vi "TRUE_Serial_GET.vi"() -> ()   [LabVIEW 2016]
uses:
  <vilib>/Instr/_visa.llb/VISA Configure Serial Port (Instr).vi
panel:
  out "Array":dbl[][](array[numeric])
  out "read buffer":string
  out "Cluster":T1
  in  "VISA resource name":refnum<visa-resource-name>
  in  "stop":bool
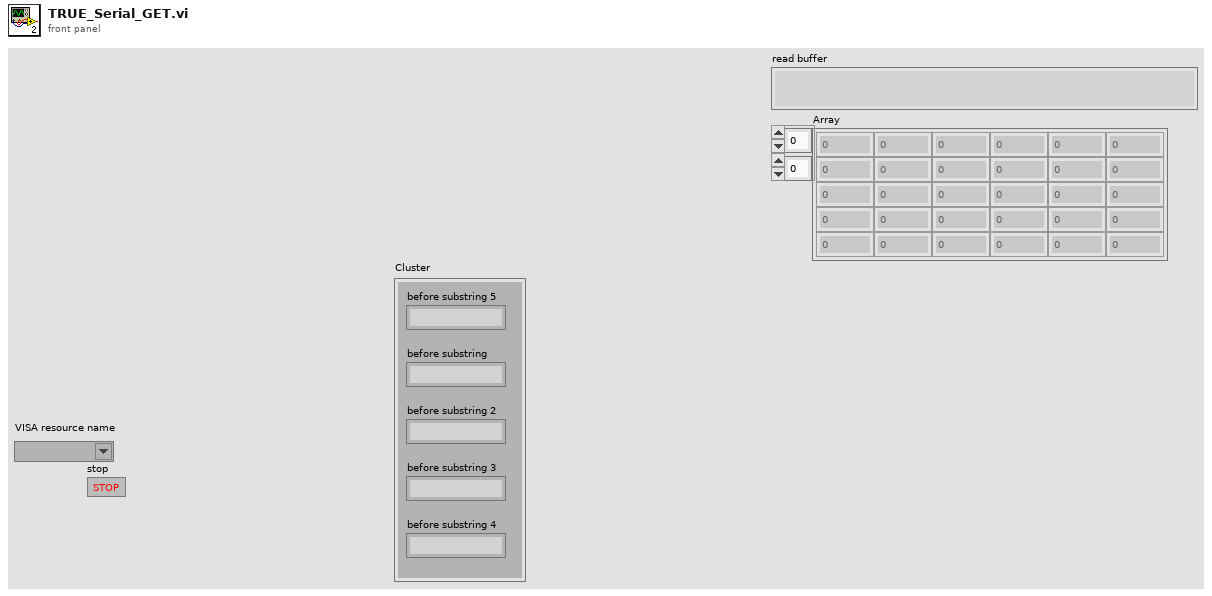
[diagram p1: front panel]
types:
  T1 = cluster{"before substring":string, "before substring 2":string, "before substring 3":string, "before substring 4":string, "before substring 5":string}
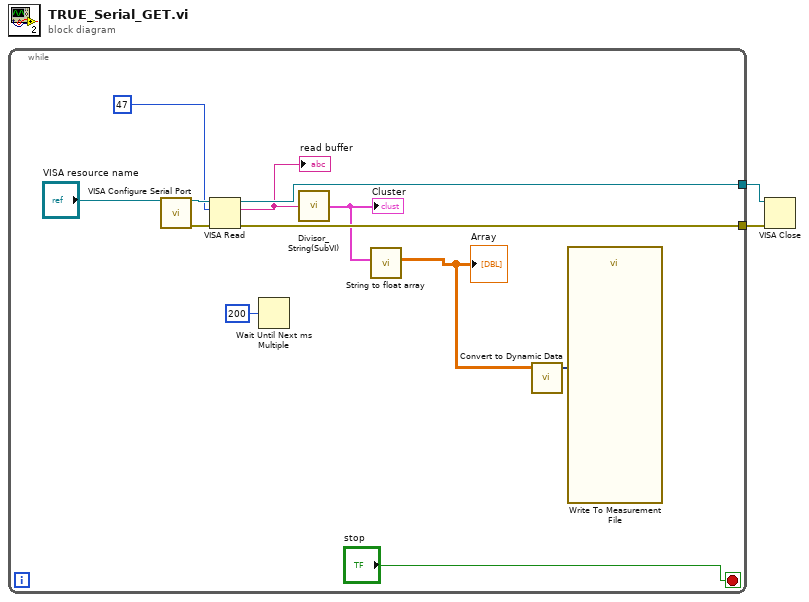
[diagram p0: block diagram]
diagram:
  n1 = while {
    tunnel: [w11] -> w2
    tunnel: [w10] -> w1
    stop <- "stop" stop-if-true
    n2 = call-poly "VISA Configure Serial Port"("VISA resource name"="VISA resource name") -> ("VISA resource name out"=w14:refnum<visa-resource-name>, "error out"=w13:errorcluster)  [unwired: 13 in]
    n3 = VISA Read(VISA resource name=w14, byte count=u32 47, error in (no error)=w13) -> (VISA resource name out=w11:refnum<visa-resource-name>, read buffer=w7:string, error out=w10:errorcluster)  [unwired: 1 out]
    "read buffer" <- w7
    n4 = Wait Until Next ms Multiple(millisecond multiple=u32 200) -> ()  [unwired: 1 out]
    n5 = call "Divisor_String(SubVI).vi"("read buffer"=w7) -> ("Cluster"=w6:T1)
    "Cluster" <- w6
    n6 = call "String to float array.vi"("Cluster"=w6) -> ("Array"=w5:dbl[][])  [unwired: 10 in]
    "Array" <- w5
    n7 = call "Convert to Dynamic Data"("2D Array"=w5) -> ("Dynamic Data Type"=w4:dynamicdata)  [unwired: 3 in]
    n8 = call "Write To Measurement File"("Signals"=w4) -> ()  [unwired: 16 in, 3 out]
  }
  n9 = VISA Close(VISA resource name=w2, error in (no error)=w1) -> ()  [unwired: 1 out]
